vi "stop_fpga.vi"(3 "error in (no error)":errorcluster, 5 "reference":refnum<visa-resource-name>) -> (0 "error out":errorcluster, 2 "VISA resource name out":refnum<visa-resource-name>)   [LabVIEW 2017]
uses:
  <vilib>/Platform/TimedLoop/XDataNode/timing_clust.ctl
  <vilib>/Platform/TimedLoop/XDataNode/nitl_modes.ctl
  <vilib>/Platform/TimedLoop/XDataNode/wakeup.ctl
  <vilib>/platform/TimedLoop/XDataNode/XDataNode.xnode
  <vilib>/Platform/TimedLoop/XDataNode/XDNodeRunTimeDep.lvlib
panel:
  out "Serial Settings:Number of Bytes at Serial Port":u32
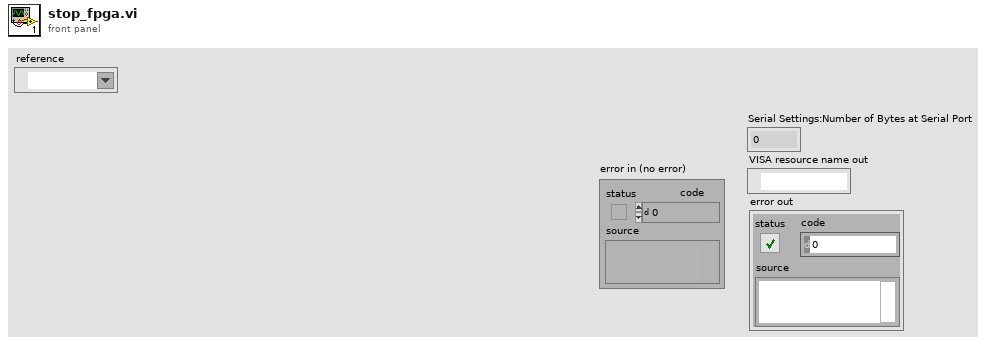
[diagram p1: front panel]
types:
  T1 = typedef "XDNodeRunTimeDep.lvlib/timing_clust.ctl" = cluster{"Expected End [f-1]":u64, "Actual End [f-1]":u64, "Finished Late? [f-1]":bool, "Expected End [i-1]":u64, "Actual End [i-1]":u64, "Finished Late? [i-1]":bool, "Expected Start [i]":u64, "Actual Start [i]":u64, "Expected Start [f]":u64, "Actual Start [f]":u64, "Source Name":string, "Structure Name":string, "Period":i64, "Deadline":i64, "Offset":i64, "Start":i64, "Priority":i32, "Timeout":i32, "Mode":T2, "Wakeup Reason":T3, "Error":errorcluster, "Source Type":string, "Secondary Source Type":string, "Global End Time":u64, "Global Start Time":u64, "Frame Duration":u64, "Iteration Duration":u64, "Assigned CPU":i32, "I/O Scan Engine Mode":u32}
  T2 = typedef "XDNodeRunTimeDep.lvlib/nitl_modes.ctl" = enum32{"No Change", "Process missed periods, maintain original phase", "Discard missed periods, maintain original phase", "Process missed periods, ignore original phase", "Discard missed periods, ignore original phase"}
  T3 = typedef "XDNodeRunTimeDep.lvlib/wakeup.ctl" = enum32{"Normal", "Aborted", "Asynchronous wakeup", "Timing source error", "Timed loop error", "Timeout"}
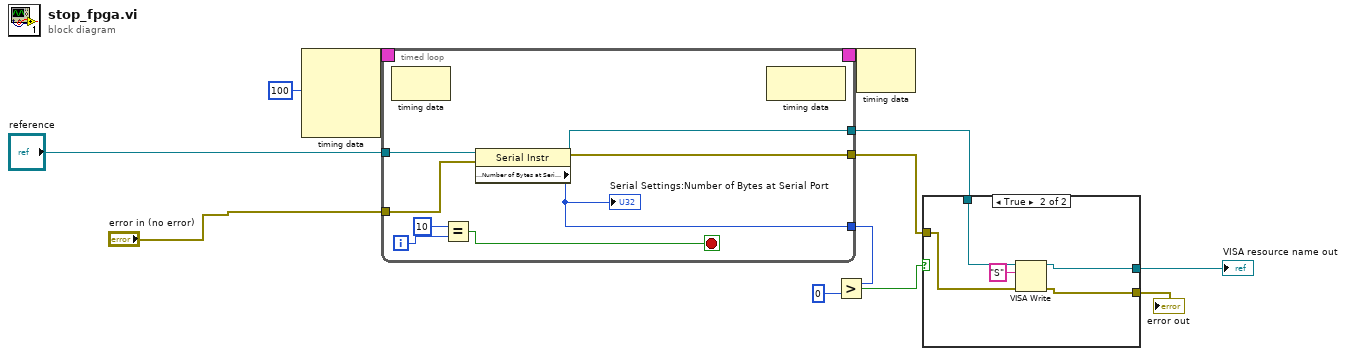
[diagram p0: block diagram]
diagram:
  n1 = node-c288(i64 100 ("Period")) -> (w12:T1)  [unwired: 3 in]
  n2 = timed-loop {
    timing: w12 -> [_]
    timing-out: [_] -> w11
    tunnel: "error in (no error)" -> [w20]
    tunnel: [w19] -> w5
    tunnel: [w18] -> w6
    tunnel: [w14] -> w8
    tunnel: "reference" -> [w13]
    i -> [w17]
    stop <- w15 stop-if-true
    n3 = node-c288() -> ()  [unwired: 1 in, 1 out]
    n4 = Equal?(x=10, y=w17) -> (x = y?=w15:bool)
    n5 = property class="Serial Instr"(reference=w13, error in=w20) -> (reference out=w18:refnum<visa-resource-name>, error out=w19:errorcluster, "Serial Settings:Number of Bytes at Serial Port"=w14:u32)
    "Serial Settings:Number of Bytes at Serial Port" <- w14
    n6 = node-c288() -> ()  [unwired: 1 in, 1 out]
  }
  n7 = Greater?(x=w8, y=u32 0) -> (0:w9:bool)
  n8 = node-c288(w11) -> ()  [unwired: 1 out]
  n9 = case shown="True" w9 {
    tunnel: w6 -> [w24 w29]
    tunnel: w5 -> [w23 w28]
    tunnel: [w23 w27] -> w3
    tunnel: [w24 w26] -> w4
    frame False {
    }
    frame True {
      n10 = VISA Write(VISA resource name=w29, write buffer="S", error in (no error)=w28) -> (VISA resource name out=w26:refnum<visa-resource-name>, error out=w27:errorcluster)  [unwired: 1 out]
    }
  }
  "VISA resource name out" <- w4
  "error out" <- w3
